vi "ObtainQueue.vi"(7 "Queue size (-1, unlimited)":i32, 8 "error in (no error)":errorcluster, 10 "Initial Message":string="Initialize", 11 "Queue Name":string) -> (0 "error out":errorcluster, 3 "MessageQueue":refnum<queue>)   [LabVIEW 2018, in "SensorPlugins.lvlib"]
doc: "This VI creates a queue based on the Queue name."
uses:
  SensorPlugins.lvlib
  clMessage.ctl
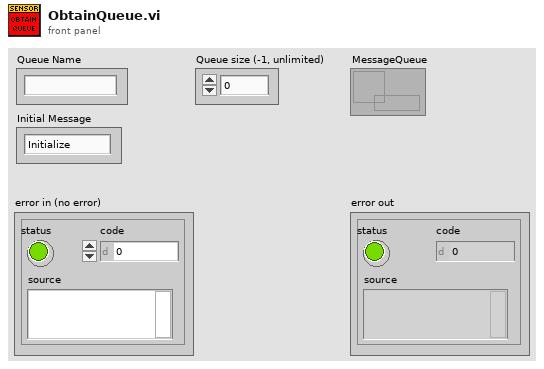
[diagram p1: front panel]
types:
  T1 = typedef "SensorPlugins.lvlib/clMessage.ctl" = cluster{"Message":string, "Message Data":variant}
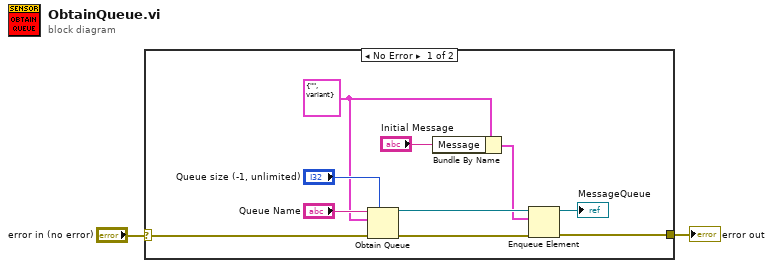
[diagram p0: block diagram]
diagram:
  n1 = case shown="No Error" "error in (no error)" {
    selector: "error in (no error)" -> [w12 w13]
    tunnel: [w8 w13] -> w1
    frame No Error {
      w4 = T1 {"Message"="", "Message Data"=variant} ("clMessage")
      n2 = Obtain Queue(max queue size (-1, unlimited)="Queue size (-1, unlimited)", name (unnamed)="Queue Name", element data type=w4, error in (no error)=w12) -> (queue out=w11:refnum<queue>, error out=w9:errorcluster)  [unwired: 1 in, 1 out]
      n3 = Bundle By Name(cluster=w4, "Message"="Initial Message") -> (w3:T1)
      n4 = Enqueue Element(queue=w11, element=w3, error in (no error)=w9) -> (queue out=→"MessageQueue":refnum<queue>, error out=w8:errorcluster)  [unwired: 1 in, 1 out]
    }
    frame Error {
    }
  }
  "error out" <- w1
